vi "Extract offset SLM.vi"(7 "current step index":i32) -> (3 "current offset":dbl)   [LabVIEW 2014]
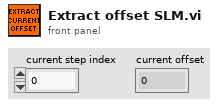
[diagram p1: front panel]
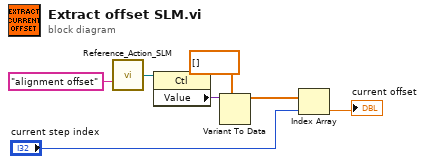
[diagram p0: block diagram]
diagram:
  n1 = call "Reference_Action_SLM.vi"("Control Name"="alignment offset") -> ("Ref OUT"=w6:refnum<vi>)  [unwired: 12 in, 2 out]
  n2 = property class="Ctl"(reference=w6) -> ("Value"=w7:variant)  [unwired: 1 in, 2 out]
  n3 = Variant To Data(type=dbl[] [], Variant=w7) -> (data=w3:dbl[])  [unwired: 1 in, 1 out]
  n4 = Index Array(array=w3, index="current step index") -> (element=→"current offset":dbl)
